vi "Check Step Condition.vi"(8 "error in (no error)":errorcluster, 9 "Postcondition?":bool, 10 "Step Number":i32, 11 "Output Sequencer in":refnum<class "Output Sequencer.lvclass">) -> (0 "error out":errorcluster, 1 "Check skipped":bool, 2 "Condition passed":bool, 3 "Output Sequencer out":refnum<class "Output Sequencer.lvclass">)   [LabVIEW 2020, in "Output Sequencer.lvlib" / "Output Sequencer.lvclass"]
uses:
  Output Sequencer.lvclass
  Output Sequencer.lvclass/Output Sequencer.ctl
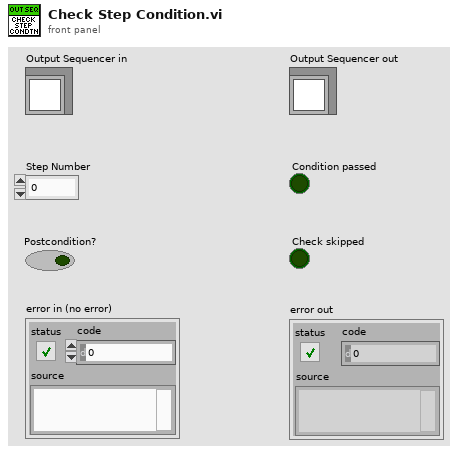
[diagram p1: front panel]
types:
  T1 = typedef "Output Sequencer.lvlib/Output Sequencer.lvclass/Compiled Step.ctl" = cluster{"Precondition":T2, "Duration":dbl, "Mode":string, "Delay Between Values":dbl, "Analog Values":T2[], "Digital Values":T2[], "Postcondition":T2, "On True":string, "On False":string}
  T2 = typedef "Output Sequencer.lvlib/Output Sequencer.lvclass/Expression Data.ctl" = cluster{"Empty?":bool, "Expression":refnum<class "mupExpr.lvclass">, "Variable Names":string[]}
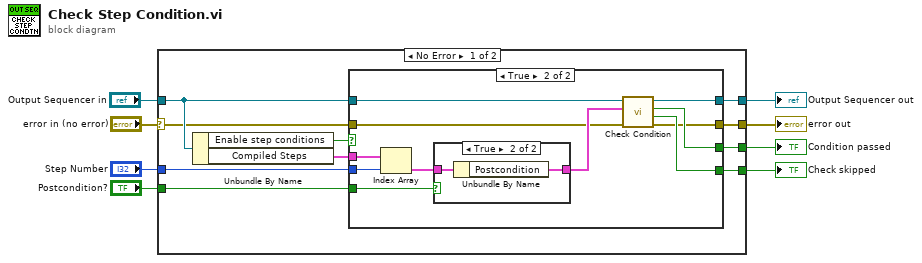
[diagram p0: block diagram]
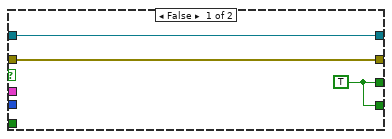
[diagram p2: hidden frame]
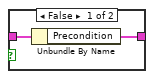
[diagram p3: hidden frame]
diagram:
  n1 = case shown="No Error" "error in (no error)" {
    selector: "error in (no error)" -> [w9 w37]
    tunnel: "Step Number" -> [w18 _]
    tunnel: "Output Sequencer in" -> [w17 w38]
    tunnel: [w16 w38] -> w6
    tunnel: [w15 _] -> w5
    tunnel: "Postcondition?" -> [w14 _]
    tunnel: [w13 _] -> w3
    tunnel: [w10 w37] -> w2
    frame No Error {
      n2 = Unbundle By Name(w17) -> ("Enable step conditions"=w11:bool, "Compiled Steps"=w12:T1[])
      n3 = case shown="True" w11 {
        tunnel: w12 -> [_ w32]
        tunnel: w18 -> [_ w31]
        tunnel: [w20 w29] -> w15
        tunnel: [w21 w28] -> w16
        tunnel: w17 -> [w21 w27]
        tunnel: w14 -> [_ w25]
        tunnel: [w20 w24] -> w13
        tunnel: w9 -> [w19 w23]
        tunnel: [w19 w22] -> w10
        frame False {
          w20 = TRUE ("Check passed")
        }
        frame True {
          n4 = Index Array(array=w32, index=w31) -> (element=w30:T1)
          n5 = case shown="True" w25 {
            tunnel: w30 -> [w34 w36]
            tunnel: [w33 w35] -> w26
            frame False {
              n6 = Unbundle By Name(w34) -> ("Precondition"=w33:T2)
            }
            frame True {
              n7 = Unbundle By Name(w36) -> ("Postcondition"=w35:T2)
            }
          }
          n8 = call "Check Condition.vi"("error in (no error)"=w23, "Expression Data"=w26, "Output Sequencer in"=w27) -> ("error out"=w22:errorcluster, "Condition empty"=w24:bool, "Check passed"=w29:bool, "Output Sequencer out"=w28:refnum<class "Output Sequencer.lvclass">)  [unwired: 5 in]
        }
      }
    }
    frame Error {
    }
  }
  "Condition passed" <- w5
  "Output Sequencer out" <- w6
  "Check skipped" <- w3
  "error out" <- w2
